vi "SetImage.vi"(8 "error in (no error)":errorcluster, 10 "Image":T1, 11 "reference in":refnum<class "Camera_IMAQdx.lvclass">) -> (0 "error out":errorcluster, 3 "reference out":refnum<class "Camera_IMAQdx.lvclass">)   [LabVIEW 2017, in "Camera_IMAQdx.lvclass"]
doc: "Gets image reference"
uses:
  Camera_IMAQdx.lvclass
  <vilib>/vision/Image Controls.llb/IMAQ Image.ctl
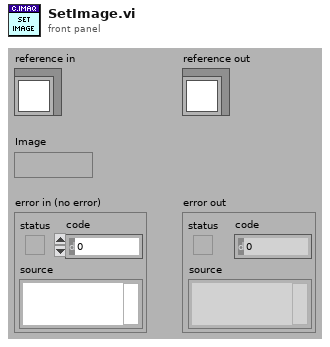
[diagram p1: front panel]
types:
  T1 = typedef "IMAQ Image.ctl" = refnum<image>
  T2 = typedef "Camera.IMAQdx.lvclass/ObjectAttributes.ctl" = cluster{"Configuration":T3, "Session":T4, "Connected":bool, "Image":T1, "Grab Frame Number":u32}
  T3 = typedef "Camera.IMAQdx.lvclass/Configuration--Cluster.ctl" = cluster{"Camera Interface Name":string, "Number of Buffers":u32, "Image Name":string}
  T4 = typedef "IMAQdx.ctl" = refnum<k21>
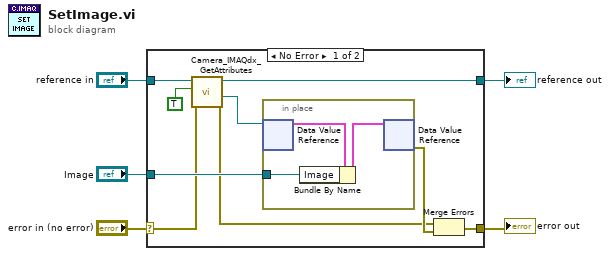
[diagram p0: block diagram]
diagram:
  n1 = case shown="No Error" "error in (no error)" {
    selector: "error in (no error)" -> [w8 w19]
    tunnel: [w12 w19] -> w4
    tunnel: [w10 w18] -> w2
    tunnel: "reference in" -> [w11 w18]
    tunnel: "Image" -> [w14 _]
    frame No Error {
      n2 = call "Camera_IMAQdx_GetAttributes.vi"("error in (no error)"=w8, "OnlyGetDvrReference(False)"=TRUE, "reference in"=w11) -> ("error out"=w7:errorcluster, "DataRef"=w9:refnum<data-value>, "reference out"=w10:refnum<class "Camera_IMAQdx.lvclass">)  [unwired: 5 in, 1 out]
      n3 = in-place {
        in-place-border: w14 -> [w17]
        n4 = in-place-dvr #1(w9) -> (w16:T2)  [unwired: 1 out]
        n5 = Bundle By Name(cluster=w16, "Image"=w17) -> (w15:T2)
        n6 = in-place-dvr #1(w15) -> (w13:errorcluster)  [unwired: 1 out]
      }
      n7 = Merge Errors(w7, w13) -> (w12:errorcluster)
    }
    frame Error {
    }
  }
  "error out" <- w4
  "reference out" <- w2
